vi "Check.vi"() -> ()   [LabVIEW 2019]
uses:
  Reg/ctl/Y_short.ctl
  Inputs/Ctl/Parameter State short.ctl
  Y_H.lvclass
  Y_H.lvclass/Y_H.ctl
  Inputs/Inputs.lvlib
  Reg/control.lvlib
panel:
  in  "input cluster":T3 {"Y_State"."Y" format="%.2f"; "Y_State"."Y_preSet" format="%.2f"; "Y_State"."SP" step=0.01 format="%.2f"; "Y_State"."Y_Set" format="%.2f"; "Y_State"."PV" step=0.01 format="%.2f"; "Y_State"."SP_Set" step=0.01 format="%.2f"}
  in  "setpoint":T4(slide) caption="oC" scale=0.0..500.0 scale format="%#_5g"
  in  "stop":bool
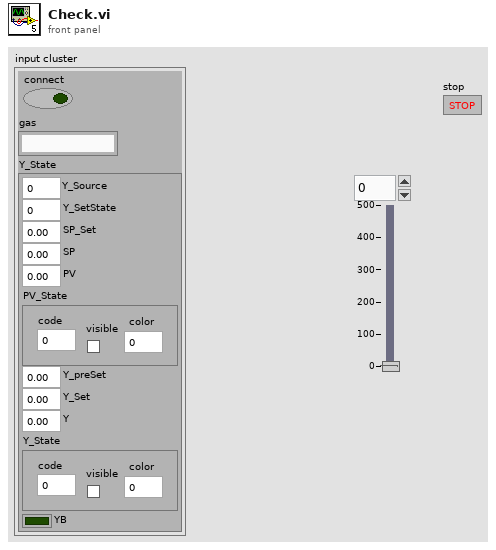
[diagram p1: front panel]
types:
  T1 = typedef "control.lvlib/Y_short.ctl" = cluster{"Y_Source":u8, "Y_SetState":u8, "SP_Set":dbl, "SP":dbl, "PV":dbl, "PV_State":T2, "Y_preSet":dbl, "Y_Set":dbl, "Y":dbl, "Y_State":T2, "YB":bool}
  T2 = typedef "Inputs.lvlib/Parameter State short.ctl" = cluster{"code":i32, "visible":bool, "color":u32}
  T3 = cluster{"connect":bool, "gas":string, "Y_State":T1}
  T4 = cluster{"Numeric":dbl, "Numeric":dbl, "Numeric":dbl}
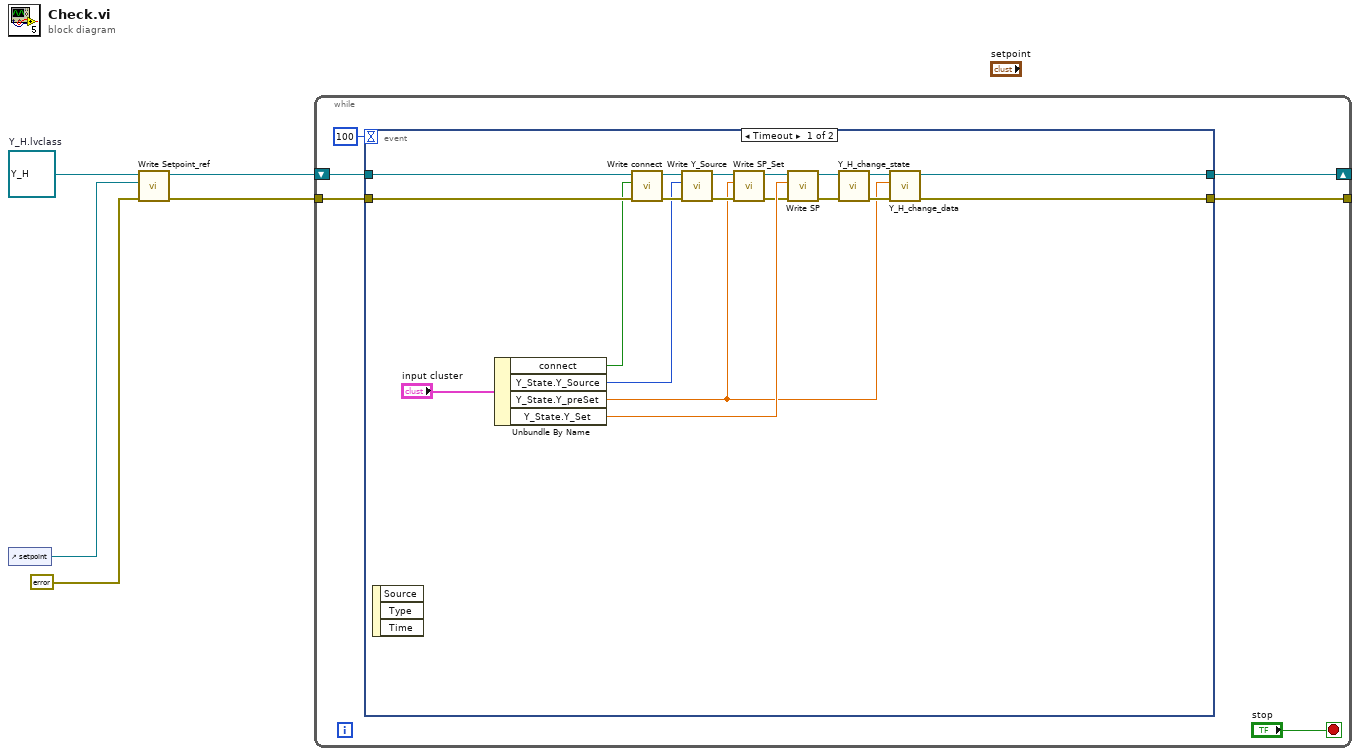
[diagram p0: block diagram]
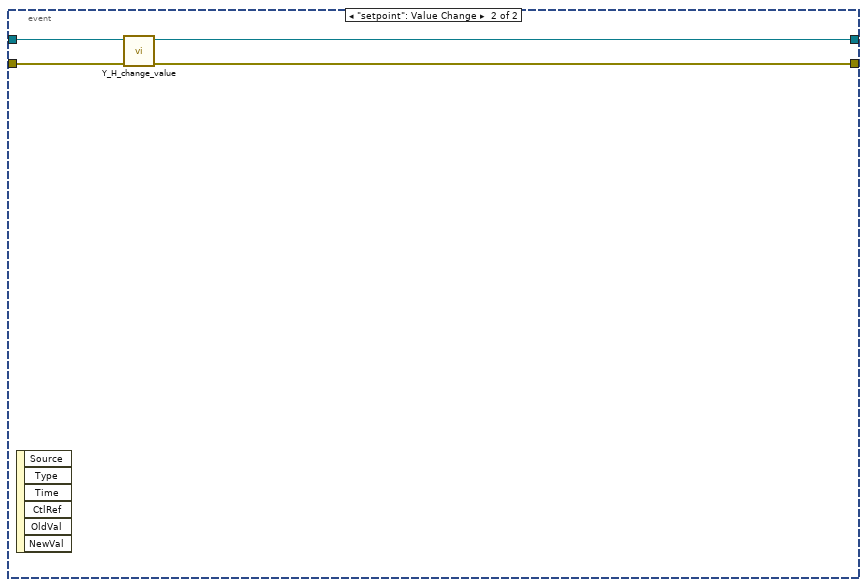
[diagram p2: hidden frame]
diagram:
  w5 = refnum<class "Y_H.lvclass"> refnum  # Y_H.lvclass
  n1 = control-ref of="setpoint"() -> (w1:refnum<vi>)
  n2 = call "Write Setpoint_ref.vi"("error in (no error)"=errorcluster {"status"=FALSE, "code"=0, "source"=""}, "setpoint ref"=w1, "Y_H in"=w5) -> ("error out"=w3:errorcluster, "Y_H out"=w4:refnum<class "Y_H.lvclass">)  [unwired: 7 in]
  n3 = while {
    tunnel: w3 -> [w7]
    shift-right: [w11] -> _
    shift-left: w4 -> [w9]
    tunnel: [w6] -> _
    stop <- "stop" stop-if-true
    n4 = event shown="[0] Timeout" {
      selector: _ -> [_ _]
      dyn-events: _ -> [_ _]
      timeout: 100 -> [_ _]
      tunnel: [w29 w32] -> w11
      tunnel: w9 -> [w28 w34]
      tunnel: w7 -> [w26 w33]
      tunnel: [w30 w31] -> w6
      event Timeout {
        n5 = event-data() -> ()  [unwired: 1 in, 3 out]
        n6 = Unbundle By Name("input cluster") -> ("connect"=w21:bool, "Y_State.Y_Source"=w20:u8, "Y_State.Y_preSet"=w12:dbl, "Y_State.Y_Set"=w19:dbl)
        n7 = call "Write connect.vi"("error in (no error)"=w26, "connect"=w21, "Y_H in"=w28) -> ("error out"=w25:errorcluster, "Y_H out"=w27:refnum<class "Y_H.lvclass">)  [unwired: 7 in]
        n8 = call "Write Y_Source.vi"("error in (no error)"=w25, "Y_Source"=w20, "Y_H in"=w27) -> ("error out"=w17:errorcluster, "Y_H out"=w18:refnum<class "Y_H.lvclass">)  [unwired: 7 in]
        n9 = call "Write SP_Set.vi"("error in (no error)"=w17, "SP_Set"=w12, "Y_H in"=w18) -> ("error out"=w15:errorcluster, "Y_H out"=w16:refnum<class "Y_H.lvclass">)  [unwired: 7 in]
        n10 = call "Write SP.vi"("error in (no error)"=w15, "SP"=w19, "Y_H in"=w16) -> ("error out"=w13:errorcluster, "Y_H out"=w14:refnum<class "Y_H.lvclass">)  [unwired: 7 in]
        n11 = call "Y_H_change_state.vi"("error in (no error)"=w13, "Y_H_in"=w14) -> ("error out"=w23:errorcluster, "Y_H_out"=w24:refnum<class "Y_H.lvclass">)  [unwired: 8 in]
        n12 = call "Y_H_change_data.vi"("error in (no error)"=w23, "SP_Set"=w12, "Y_H_in"=w24) -> ("error out"=w30:errorcluster, "Y_H_out"=w29:refnum<class "Y_H.lvclass">)  [unwired: 7 in]
      }
      event "setpoint": Value Change {
        n13 = event-data() -> ()  [unwired: 1 in, 6 out]
        n14 = call "Y_H_change_value.vi"("error in (no error)"=w33, "Y_H_in"=w34) -> ("error out"=w31:errorcluster, "Y_H_out"=w32:refnum<class "Y_H.lvclass">)  [unwired: 8 in]
      }
    }
  }
